vi "Read Write Data.vi"(7 "Command":T2, 8 "error in (no error)":errorcluster, 10 "Array In":T1(array[cluster]), 11 "file path":path) -> (0 "error IO":errorcluster, 2 "Array out":T1(array[cluster]))   [LabVIEW 2013]
doc: "This subVI is used to-\n-Initialize the file path.\n-Reads the data from provided file path.\n-Writes the data to the provided file path.\n-Release the file path."
uses:
  Controls/Read Write States.ctl
  <vilib>/Utility/file.llb/Read From Spreadsheet File (string).vi
  <vilib>/Utility/file.llb/Write To Spreadsheet File (string).vi
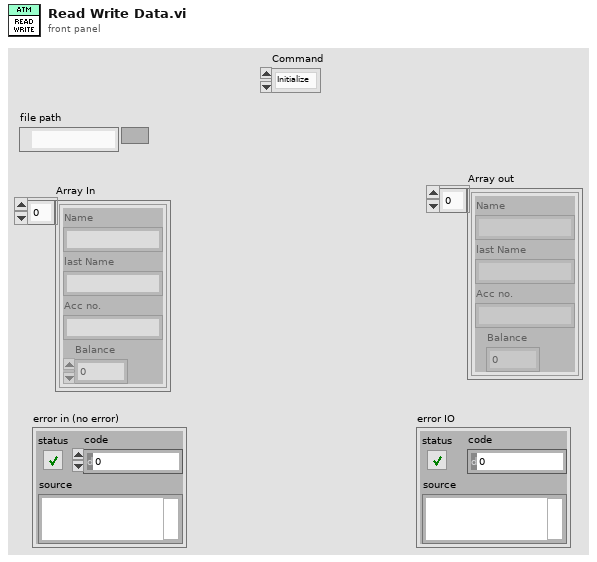
[diagram p1: front panel]
types:
  T1 = cluster{"Name":string, "last Name":string, "Acc no.":string, "Balance":i32}[]
  T2 = typedef "Read Write States.ctl" = enum16{"Initialize", "Read Data ", "Write Data", "Stop"}
  T3 = cluster{"Name":string, "Company":string, "Acc no.":string, "Balance":i32}[]
  T4 = cluster{"Name":string, "Last Name":string, "Acc no.":string, "Balance":i32}
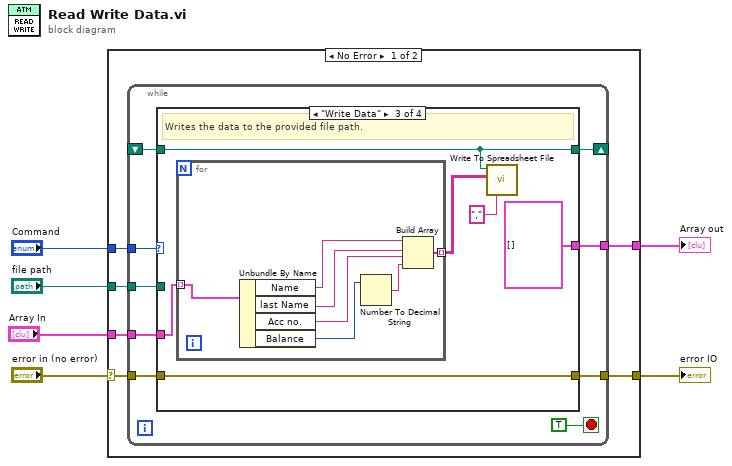
[diagram p0: block diagram]
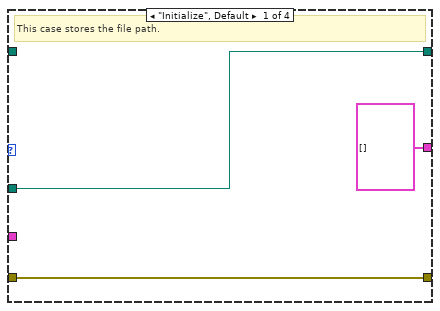
[diagram p2: hidden frame]
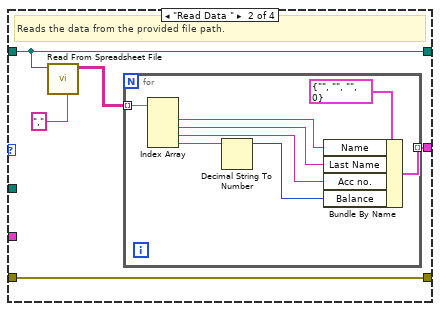
[diagram p3: hidden frame]
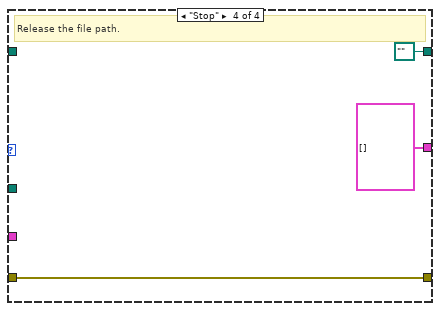
[diagram p4: hidden frame]
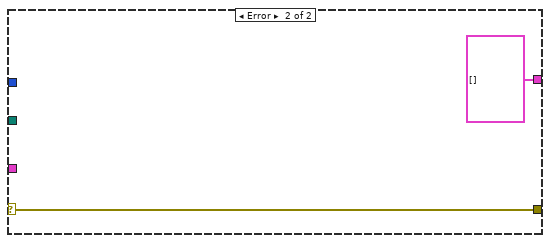
[diagram p5: hidden frame]
diagram:
  n1 = case shown="No Error" "error in (no error)" {
    selector: "error in (no error)" -> [w9 w55]
    tunnel: "Command" -> [w12 _]
    tunnel: "file path" -> [w11 _]
    tunnel: [w10 T3 []] -> w5
    tunnel: [w8 w55] -> w2
    tunnel: "Array In" -> [w7 _]
    frame No Error {
      n2 = while {
        tunnel: w12 -> [w20]
        tunnel: w11 -> [w19]
        shift-right: [w18] -> _
        shift-left: _ -> [w17]
        tunnel: [w16] -> w10
        tunnel: w9 -> [w15]
        tunnel: [w14] -> w8
        tunnel: w7 -> [w13]
        stop <- TRUE stop-if-true
        n3 = case shown="\"Write Data\"" w20 {
          tunnel: w19 -> [w24 _ _ _]
          tunnel: [w24 w29 w43 path "" ("file path")] -> w18
          tunnel: w17 -> [_ w29 w43 _]
          tunnel: [T3 [] w26 T3 [] T3 []] -> w16
          tunnel: w15 -> [w22 w25 w41 w51]
          tunnel: [w22 w25 w41 w51] -> w14
          tunnel: w13 -> [_ _ w39 _]
          frame "Initialize", Default {
            # "This case stores the file path."
          }
          frame "Read Data " {
            # "Reads the data from the provided file path."
            n4 = call-poly <vilib>:"Read From Spreadsheet File.vi"("delimiter (\\t)"="," ("delimiter (\\t)"), "file path (dialog if empty)"=w29) -> ("all rows"=w27:string[][])  [unwired: 5 in, 4 out]
            n5 = for {
              tunnel: w27 -> [w37] mode=indexing
              tunnel: [w36] -> w26 mode=indexing
              n6 = Index Array(array=w37) -> (element #1=w34:string, element #2=w33:string, element #3=w32:string, element #4=w31:string)  [unwired: 4 in]
              n7 = Decimal String To Number(string=w31) -> (number=w30:i32)  [unwired: 2 in, 1 out]
              n8 = Bundle By Name(cluster=T4 {"Name"="", "Last Name"="", "Acc no."="", "Balance"=0} ("data In  2"), "Name"=w34, "Last Name"=w33, "Acc no."=w32, "Balance"=w30) -> (w36:T4)
            }
          }
          frame "Write Data" {
            # "Writes the data to the provided file path."
            n9 = for {
              tunnel: w39 -> [w44] mode=indexing
              tunnel: [w45] -> w38 mode=indexing
              n10 = Unbundle By Name(w44) -> ("Name"=w50:string, "last Name"=w49:string, "Acc no."=w48:string, "Balance"=w46:i32)
              n11 = Number To Decimal String(number=w46) -> (decimal integer string=w47:string)  [unwired: 1 in]
              n12 = Build Array(w50, w49, w48, w47) -> (w45:string[])
            }
            n13 = call-poly <vilib>:"Write To Spreadsheet File.vi"("delimiter (\\t)"="," ("delimiter (\\t)"), "2D data"=w38, "file path (dialog if empty)"=w43) -> ()  [unwired: 5 in, 1 out]
          }
          frame "Stop" {
            # "Release the file path."
          }
        }
      }
    }
    frame Error {
    }
  }
  "Array out" <- w5
  "error IO" <- w2
